vi "Handle path to LUT.vi"(8 "error in (no error)":errorcluster, 11 "Path to LUT":path=path "C:/Program Files (x86)/National Instruments/LabVIEW 2017/instr.lib/ANC350/ANRv51-C4-124.LUT") -> (0 "error out":errorcluster, 3 "LUT path out":path=path "C:/Program Files (x86)/National Instruments/LabVIEW 2017/instr.lib/ANC350/Win64/anc350v4.dll")   [LabVIEW 2022 SP3, in "SampleRotator.lvlib"]
uses:
  SampleRotator.lvlib
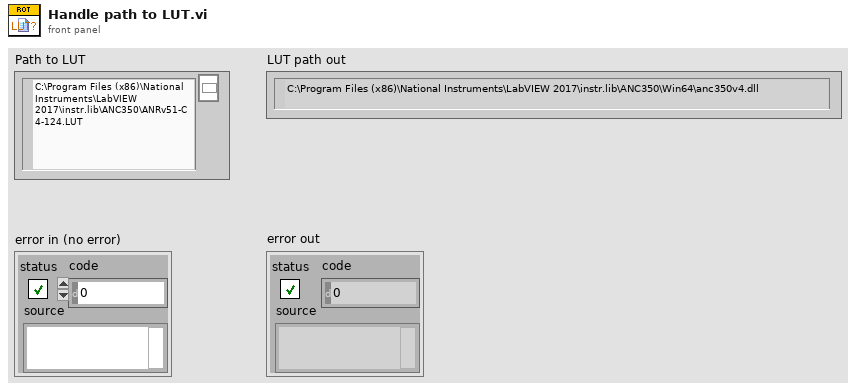
[diagram p1: front panel]
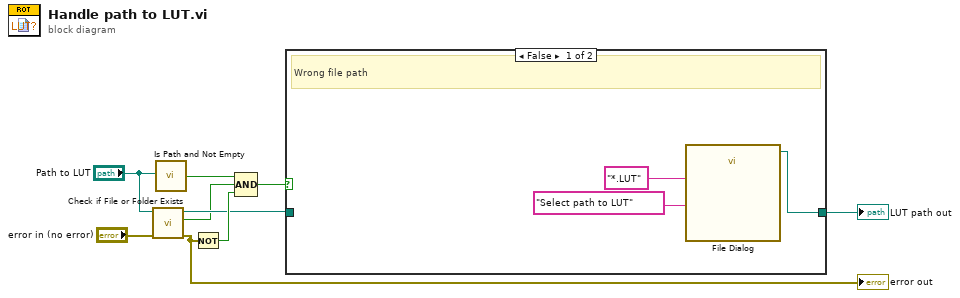
[diagram p0: block diagram]
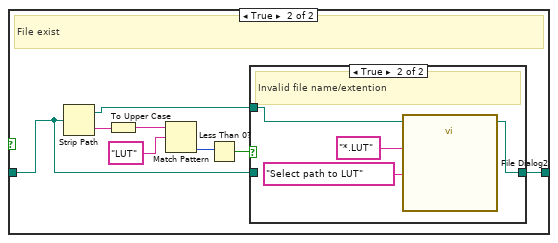
[diagram p2: hidden frame]
diagram:
  n1 = call <vilib>:"Check if File or Folder Exists.vi"("error in (no error)"="error in (no error)", "path"="Path to LUT") -> ("error out"=w8:errorcluster, "file or folder exists?"=w3:bool, "dup path"=w5:path)  [unwired: 7 in]
  "error out" <- w8
  n2 = call <vilib>:"Is Path and Not Empty.vi"("path"="Path to LUT") -> ("Is Path and Not Empty?"=w2:bool)  [unwired: 4 in]
  n3 = Not(x=w8) -> (.not. x?=w9:bool)
  n4 = Compound Arithmetic op=AND(w2, w3, w9) -> (w4:bool)
  n5 = case shown="False" w4 {
    tunnel: w5 -> [_ w13]
    tunnel: [w10 w16] -> w6
    frame False {
      # "Wrong file path"
      n6 = call "File Dialog"("prompt"="Select path to LUT", "pattern (all files)"="*.LUT") -> ("selected path"=w10:path)  [unwired: 10 in, 3 out]
    }
    frame True {
      # "File exist"
      n7 = Strip Path(path=w13) -> (stripped path=w15:path, name=w20:string)
      n8 = To Upper Case(1:w20) -> (0:w19:string)
      n9 = Match Pattern(string=w19, regular expression="LUT") -> (offset past match=w17:i32)  [unwired: 1 in, 3 out]
      n10 = Less Than 0?(x=w17) -> (x < 0?=w14:bool)
      n11 = case shown="True" w14 {
        tunnel: [w21 w23] -> w16
        tunnel: w15 -> [_ w22]
        tunnel: w13 -> [w21 _]
        frame False {
          # "File contains \"LUT\" in it's name"
        }
        frame True {
          # "Invalid file name/extention"
          n12 = call "File Dialog2"("start path"=w22, "prompt"="Select path to LUT", "pattern (all files)"="*.LUT") -> ("selected path"=w23:path)  [unwired: 9 in, 3 out]
        }
      }
    }
  }
  "LUT path out" <- w6
